vi "ROI - Fill Tree.vi"(0 "TreeControl in":refnum<vi>, 5 "ROIs":T1[](array[typedef]) {"Type" items=["Point", "Line", "Rectangle", "Oval", "Freehand / Polygon"]}, 11 "error in (no error)":errorcluster) -> (4 "TreeControl out":refnum<vi>, 6 "Active Item Row Number":dbl, 15 "error out":errorcluster)   [LabVIEW 2014]
doc: "Used to fill a tree element with ROI data"
uses:
  MSC Image_class/controls/ROI.ctl
  MSC Image_class/controls/ROI Type.ctl
  MSC Image_class/controls/Contour.ctl
  MSC Image_class/controls/Contour hierarchy.ctl
  <userlib>/MSC-Tree/SW Code/Tree -string-/sub VIs/spring action.ctl
  MSC Image_class/MSC Image.lvclass
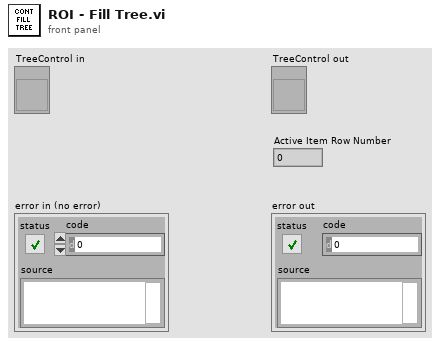
[diagram p1: front panel]
types:
  T1 = typedef "MSC Image.lvclass/ROI.ctl" = cluster{"Type":T2, "Parameters":dbl[], "Contour":T3, "Bounding Box":T3, "Contour Length":dbl, "ROI Area":dbl, "ROI Mean":dbl, "ROI Standard Deviation":dbl, "ROI Min":dbl, "ROI Max":dbl, "Hierarchy":T4, "Variant":variant, "Timestamp":timestamp}
  T2 = typedef "MSC Image.lvclass/ROI Type.ctl" = u16
  T3 = typedef "MSC Image.lvclass/Contour.ctl" = cluster{"x":i16, "y":i16}[]
  T4 = typedef "MSC Image.lvclass/Contour hierarchy.ctl" = cluster{"parent ID":i32, "children IDs":dbl[], "level":i32}
  T5 = typedef "spring action.ctl" = enum16{"_init", "_add tree", "set itemstrings", "set fg colors", "set bg colors", "set symbols", "get tags", "get itemstrings", "get fg colors", "get bg colors", "get symbols", "empty tree", "update from tree"}
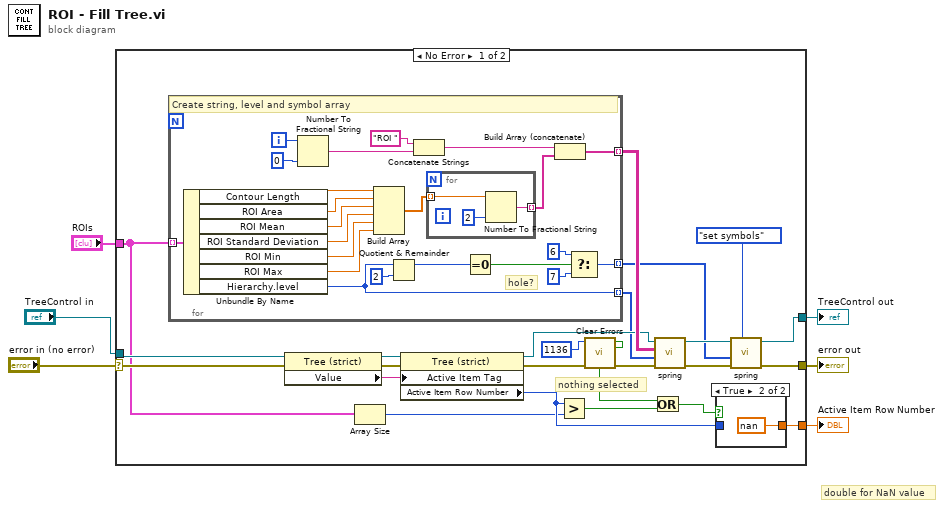
[diagram p0: block diagram]
diagram:
  # "double for NaN value"
  n1 = case shown="No Error" "error in (no error)" {
    selector: "error in (no error)" -> [w20 w59]
    tunnel: [w19 _] -> w6
    tunnel: [w27 w59] -> w5
    tunnel: [w26 w58] -> w4
    tunnel: "ROIs" -> [w18 _]
    tunnel: "TreeControl in" -> [w21 w58]
    frame No Error {
      # "nothing selected"
      n2 = for {
        tunnel: w18 -> [w54] mode=indexing
        tunnel: [w43] -> w22 mode=indexing
        tunnel: [w34] -> w13 mode=indexing
        tunnel: [w33] -> w12 mode=indexing
        i -> [w46]
        # "hole?"
        # "Create string, level and symbol array"
        n3 = Unbundle By Name(w54) -> ("Contour Length"=w53:dbl, "ROI Area"=w52:dbl, "ROI Mean"=w51:dbl, "ROI Standard Deviation"=w50:dbl, "ROI Min"=w49:dbl, "ROI Max"=w48:dbl, "Hierarchy.level"=w34:i32)
        n4 = Number To Fractional String(number=w46, precision (6)=i16 0) -> (F-format string=w42:string)  [unwired: 2 in]
        n5 = Build Array(w53, w52, w51, w50, w49, w48) -> (w47:dbl[])
        n6 = Quotient & Remainder(x=w34, y=2 ("Numeric")) -> (x-y*floor(x/y)=w38:i32)  [unwired: 1 out]
        n7 = Concatenate Strings("ROI " ("string"), w42) -> (w41:string)
        n8 = for {
          tunnel: w47 -> [w57] mode=indexing
          tunnel: [w55] -> w44 mode=indexing
          n9 = Number To Fractional String(number=w57, precision (6)=i16 2) -> (F-format string=w55:string)  [unwired: 2 in]
        }
        n10 = Equal To 0?(x=w38) -> (x = 0?=w39:bool)
        n11 = Build Array (concatenate)(w41, w44) -> (w43:string[])
        n12 = Select(t=6, s=w39, f=7) -> (s? t:f=w33:i32)
      }
      n13 = property class="Tree (strict)"(reference=w21, error in=w20) -> (reference out=w28:refnum<vi>, error out=w29:errorcluster, "Value"=w30:string)
      n14 = Array Size(array=w18) -> (size(s)=w14:i32)
      n15 = property on="Property Node" class="Tree (strict)"(reference=w28, error in=w29, "Active Item Tag"=w30) -> (reference out=w17:refnum<vi>, error out=w9:errorcluster, "Active Item Row Number"=w15:i32)
      n16 = Greater?(x=w15, y=w14) -> (0:w11:bool)
      n17 = call <vilib>:"Clear Errors.vi"("error in (no error)"=w9, "specific error code to clear (0: all)"=1136 ("error code")) -> ("error out"=w8:errorcluster, "specific error cleared?"=w7:bool)  [unwired: 4 in]
      n18 = Or(x=w7, y=w11) -> (x .or. y?=w16:bool)
      n19 = call <userlib>:"spring.vi"("error in (no error)"=w8, "indentation/item symbols/colors in"=w13, "item strings in"=w22, "tree RefNum in"=w17) -> ("error out"=w23:errorcluster, "dup tree RefNum"=w24:refnum<vi>)  [unwired: 4 in, 2 out]
      n20 = case shown="True" w16 {
        tunnel: [w31 nan] -> w19
        tunnel: w15 -> [w31 _]
        frame False {
        }
        frame True {
        }
      }
      n21 = call <userlib>:"spring.vi"("action (set itemstrings)"=spring_action."set symbols", "error in (no error)"=w23, "indentation/item symbols/colors in"=w12, "tree RefNum in"=w24) -> ("error out"=w27:errorcluster, "dup tree RefNum"=w26:refnum<vi>)  [unwired: 4 in, 2 out]
    }
    frame Error {
    }
  }
  "Active Item Row Number" <- w6
  "error out" <- w5
  "TreeControl out" <- w4
